vi "Cursor Unset Busy.vi"(8 "error in (no error)":errorcluster, 11 "LF2R IDE in":refnum<class "Main Panel.lvclass">) -> (0 "error out":errorcluster, 3 "LF2R IDE out":refnum<class "Main Panel.lvclass">)   [LabVIEW 2018, in "Main Panel.lvlib" / "Main Panel.lvclass"]
uses:
  Main Panel.lvclass
  Main Panel.lvclass/Main Panel.ctl
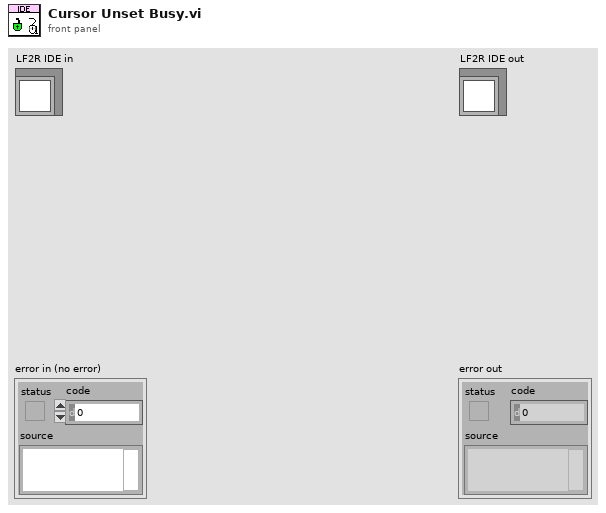
[diagram p1: front panel]
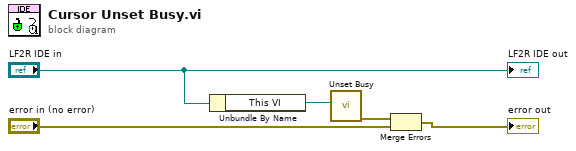
[diagram p0: block diagram]
diagram:
  n1 = Unbundle By Name("LF2R IDE in") -> ("This VI"=w2:refnum<vi>)
  n2 = call <vilib>:"Unset Busy.vi"("VI reference (current VI)"=w2) -> ("error out"=w1:errorcluster)  [unwired: 10 in]
  n3 = Merge Errors(w1, "error in (no error)") -> (→"error out":errorcluster)
  "LF2R IDE out" <- "LF2R IDE in"
